vi "DAQ.VR.Read.vi"(8 "error in (no error)":errorcluster, 11 "DAQ.Virtual in":refnum<class "DAQ.Virtual.lvclass">) -> (0 "error out":errorcluster, 2 "Waveforms":T1, 3 "DAQ.Virtual out":refnum<class "DAQ.Virtual.lvclass">)   [LabVIEW 2016, in "DAQ.Virtual.lvclass"]
uses:
  DAQ.Virtual.lvclass
  DAQ/Typedefs/PublicEvents--DAQ.Read.ctl
  <vilib>/measure/NI_MABase.lvlib
  DAQ/DAQ.lvclass
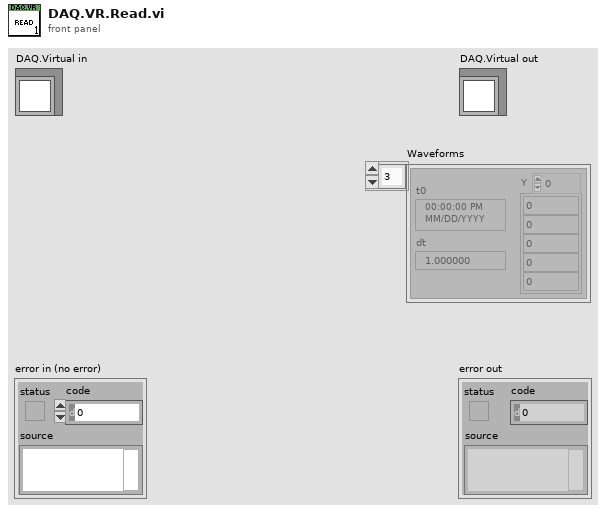
[diagram p1: front panel]
types:
  T1 = typedef "DAQ.lvclass/PublicEvents--DAQ.Read.ctl" = waveform(dbl)[]
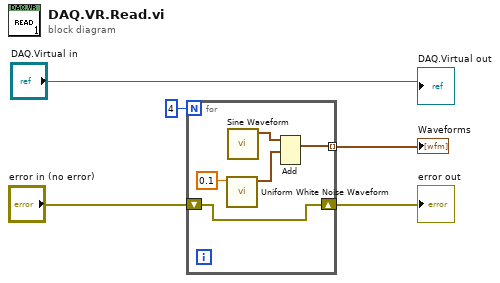
[diagram p0: block diagram]
diagram:
  n1 = for {
    N: 4 -> [_]
    tunnel: [w10] -> w5 mode=indexing
    shift-right: [w6] -> w2
    shift-left: "error in (no error)" -> [w6]
    n2 = call <vilib>:"Uniform White Noise Waveform.vi"("amplitude"=0.1) -> ("signal out"=w8:waveform(dbl))  [unwired: 9 in, 1 out]
    n3 = call <vilib>:"Sine Waveform.vi"() -> ("signal out"=w9:waveform(dbl))  [unwired: 10 in, 1 out]
    n4 = Add(1:w8, 2:w9) -> (0:w10:waveform(dbl))  [unwired: 1 in, 1 out]
  }
  "error out" <- w2
  "Waveforms" <- w5
  "DAQ.Virtual out" <- "DAQ.Virtual in"
